vi "Clear Bindings.vi"(8 "error in (no error)":errorcluster, 11 "SQL Statement in":refnum<class "SQL Statement.lvclass">) -> (0 "error out":errorcluster, 2 "Unused":bool, 3 "SQL Statement out":refnum<class "SQL Statement.lvclass">)   [LabVIEW 2023, in "SQLiteSupport.lvlib" / "SQL Statement.lvclass"]
doc: "Sets all parameter bindings to NULL and resets the Next Bind to zero. \n\nNote that \"Reset.vi\" does not clear the previously bound parameters.\n\nNo input is needed; an unused output is provided for compatability as a property node."
uses:
  SQL Statement.lvclass
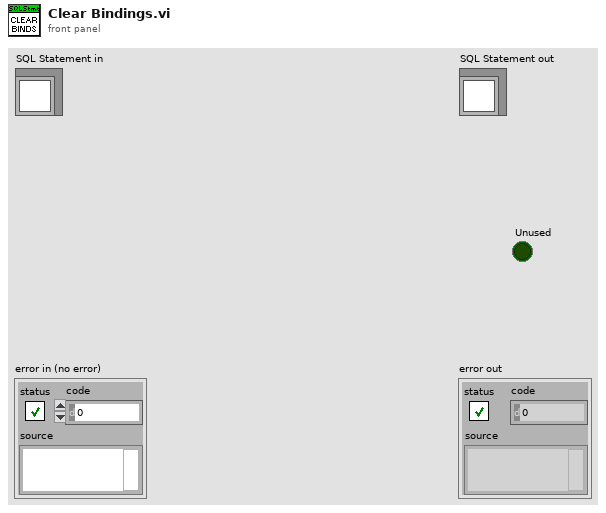
[diagram p1: front panel]
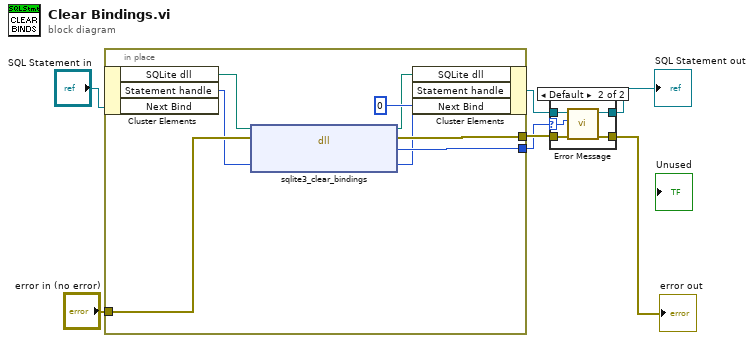
[diagram p0: block diagram]
diagram:
  n1 = in-place {
    in-place-border: "error in (no error)" -> [w15]
    in-place-border: [w14] -> w6
    in-place-border: [w13] -> w5
    n2 = in-place-cluster #1("SQL Statement in") -> ("SQLite dll"=w12:path, "Statement handle"=w8:u64)  [unwired: 1 out]
    n3 = dll-call lib="C:/LabVIEW_JDP/Support/SQLite/sqlite3.dll" fn="sqlite3_clear_bindings"(path in=w12, error in=w15, "Statement"=w8) -> (path out=w10:path, error out=w14:errorcluster, "Result Code"=w13:i32, "Statement"=w9:u64)  [unwired: 1 in]
    n4 = in-place-cluster #1("SQLite dll"=w10, "Statement handle"=w9, "Next Bind"=0) -> (w1:refnum<class "SQL Statement.lvclass">)
  }
  n5 = case shown="Default" w5 {
    selector: w5 -> [_ w18]
    tunnel: w1 -> [w17 w22]
    tunnel: [w17 w21] -> w4
    tunnel: w6 -> [w16 w20]
    tunnel: [w16 w19] -> w3
    frame 0 {
      # "No Error"
    }
    frame Default {
      n6 = call "Error Message.vi"("error in (no error)"=w20, "error code"=w18, "SQL Statement In"=w22) -> ("error out"=w19:errorcluster, "SQL Statement Out"=w21:refnum<class "SQL Statement.lvclass">)  [unwired: 7 in]
    }
  }
  "error out" <- w3
  "SQL Statement out" <- w4
